vi "setTuning.vi"(0 "Interface in":T4, 5 "TuningParameters":T1 {"gains"."proportional gain" step=0.125}, 11 "error in (no error)":errorcluster) -> (4 "Interface out":T4, 15 "error out":errorcluster)   [LabVIEW 2017, in "BuckBoostInterface.lvlib"]
uses:
  BuckBoostInterface.lvlib
  Interface.ctl
  <instrlib>/_niInstr/Instruction Framework/v1/Host/Instruction Target/niInstr Instruction Target v1 Host.lvclass
  <instrlib>/_niInstr/Instruction Framework/v1/Host/Instruction Framework Context/niInstr Instruction Framework Context v1 Host.lvclass
  TuningParameters.ctl
  <vilib>/rvi/Analysis/control/PID/Typedef/niFpgaPID_PIGains.ctl
  FPGA/contState.ctl
  FPGA/BuckBoost.lvlib
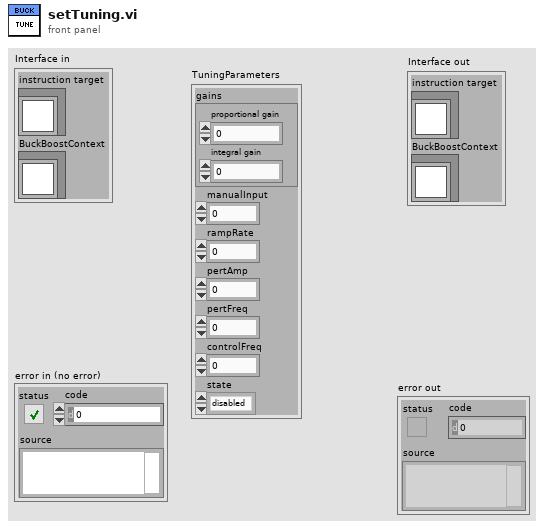
[diagram p1: front panel]
types:
  T1 = typedef "BuckBoostInterface.lvlib/TuningParameters.ctl" = cluster{"gains":T2, "manualInput":sgl, "rampRate":sgl, "pertAmp":sgl, "pertFreq":sgl, "controlFreq":sgl, "state":T3}
  T2 = typedef "niFpgaPID_PIGains.ctl" = cluster{"proportional gain":sgl, "integral gain":sgl}
  T3 = typedef "BuckBoost.lvlib/contState.ctl" = enum16{"disabled", "manual", "normal", "perturb"}
  T4 = typedef "BuckBoostInterface.lvlib/Interface.ctl" = cluster{"instruction target":refnum<class "niInstr Instruction Target v1 Host.lvclass">, "BuckBoostContext":refnum<class "niInstr Instruction Framework Context v1 Host.lvclass">}
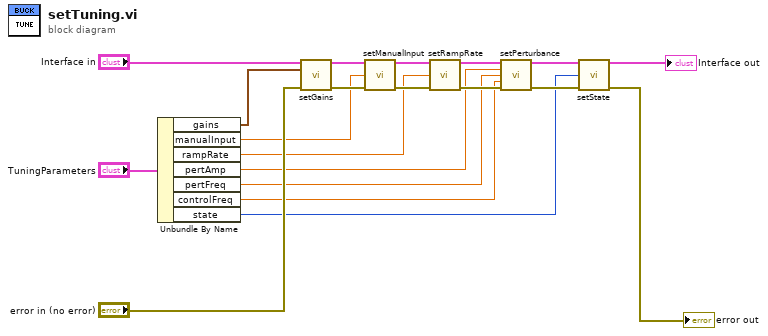
[diagram p0: block diagram]
diagram:
  n1 = Unbundle By Name("TuningParameters") -> ("gains"=w7:T2, "manualInput"=w6:sgl, "rampRate"=w5:sgl, "pertAmp"=w4:sgl, "pertFreq"=w3:sgl, "controlFreq"=w2:sgl, "state"=w1:T3)
  n2 = call "setGains.vi"("Interface in"="Interface in", "gains"=w7, "error in (no error)"="error in (no error)") -> ("Interface out"=w19:T4, "error out"=w18:errorcluster)  [unwired: 11 in]
  n3 = call "setManualInput.vi"("Interface in"=w19, "manualInput"=w6, "error in (no error)"=w18) -> ("Interface out"=w17:T4, "error out"=w16:errorcluster)  [unwired: 11 in]
  n4 = call "setRampRate.vi"("Interface in"=w17, "rampRate"=w5, "error in (no error)"=w16) -> ("Interface out"=w15:T4, "error out"=w14:errorcluster)  [unwired: 11 in]
  n5 = call "setPerturbance.vi"("Interface in"=w15, "pertAmp"=w4, "pertFreq"=w3, "controlFreq"=w2, "error in (no error)"=w14) -> ("Interface out"=w13:T4, "error out"=w12:errorcluster)  [unwired: 9 in]
  n6 = call "setState.vi"("Interface in"=w13, "state"=w1, "error in (no error)"=w12) -> ("Interface out"=→"Interface out":T4, "error out"=→"error out":errorcluster)  [unwired: 11 in]
